vi "Read CurrentLastSetpoint.vi"(8 "error in (no error)":errorcluster, 11 "RMXPowerSupply in":refnum<class "RMXPowerSupply.lvclass">) -> (0 "error out":errorcluster, 2 "CurrentLastSetpoint":dbl, 3 "RMXPowerSupply out":refnum<class "RMXPowerSupply.lvclass">)   [LabVIEW 2023, in "RMXPowerSupply.lvclass"]
uses:
  RMXPowerSupply.lvclass
  RMXPowerSupply.lvclass/RMXPowerSupply.ctl
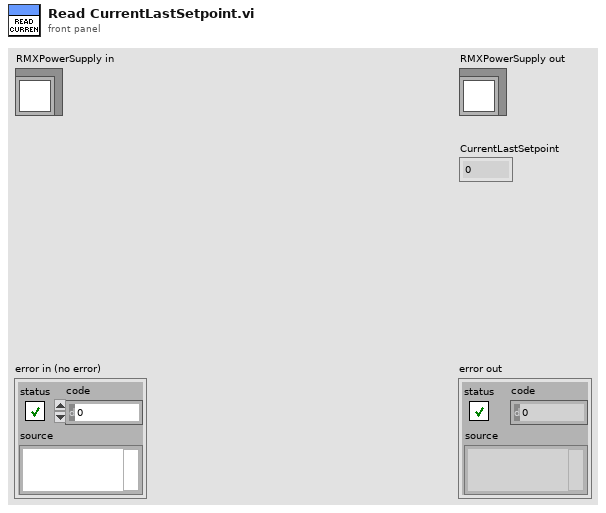
[diagram p1: front panel]
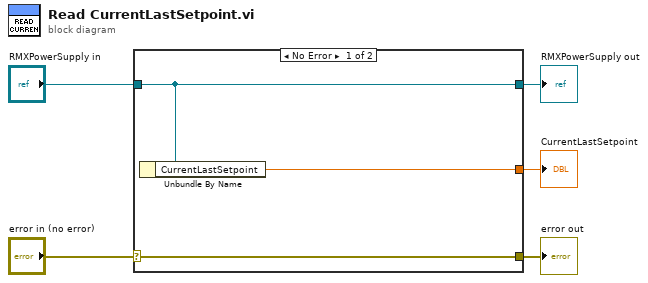
[diagram p0: block diagram]
diagram:
  n1 = case shown="No Error" "error in (no error)" {
    selector: "error in (no error)" -> [w8 w9]
    tunnel: [w8 w9] -> w4
    tunnel: [w7 w10] -> w2
    tunnel: "RMXPowerSupply in" -> [w7 w10]
    tunnel: [w6 _] -> w1
    frame No Error {
      n2 = Unbundle By Name(w7) -> ("CurrentLastSetpoint"=w6:dbl)
    }
    frame Error {
    }
  }
  "error out" <- w4
  "RMXPowerSupply out" <- w2
  "CurrentLastSetpoint" <- w1
